vi "ActionController.vi"(0 "Error In":errorcluster, 5 "Water":dbl, 7 "Sound":dbl, 9 "on/off toggle":bool, 11 "direction toggle 2":bool) -> (4 "Error Out":errorcluster, 6 "감속":bool, 8 "LCD 변경":bool)   [LabVIEW 2019]
uses:
  LINE_2.vi
  LINE_1.vi
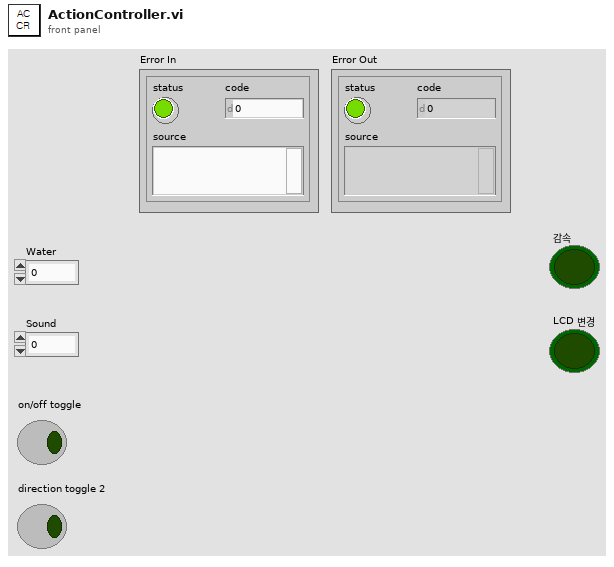
[diagram p1: front panel]
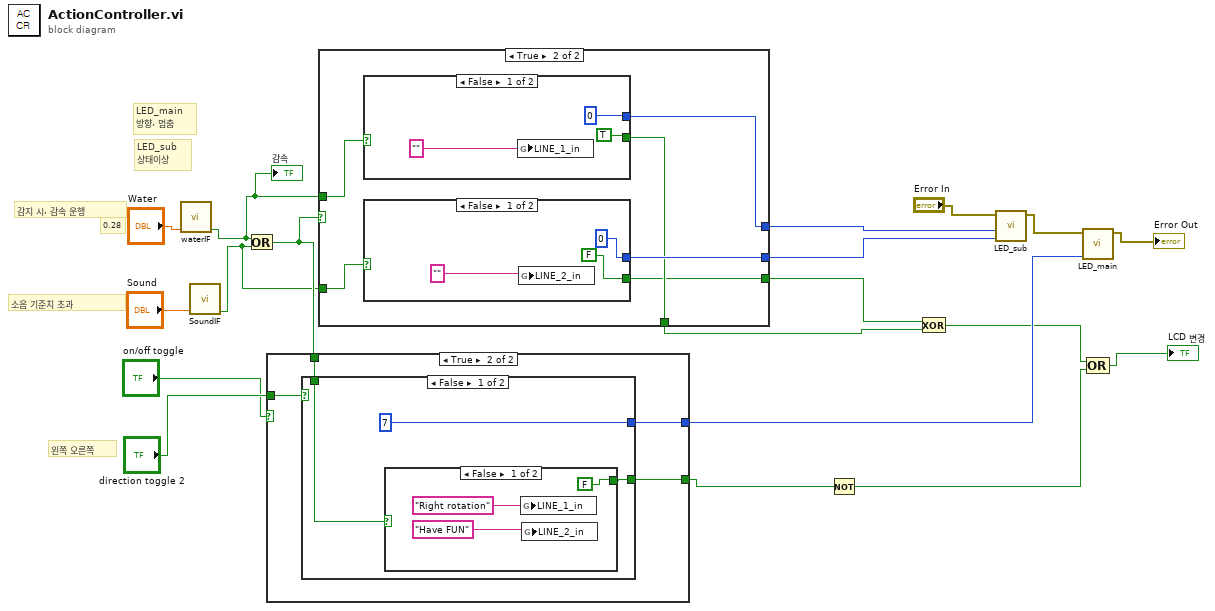
[diagram p0: block diagram]
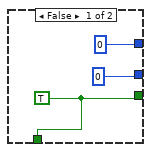
[diagram p2: hidden frame]
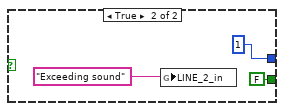
[diagram p3: hidden frame]
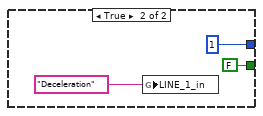
[diagram p4: hidden frame]
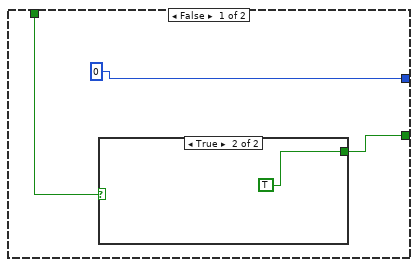
[diagram p5: hidden frame]
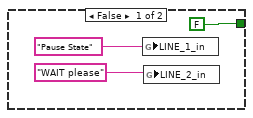
[diagram p6: hidden frame]
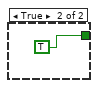
[diagram p7: hidden frame]
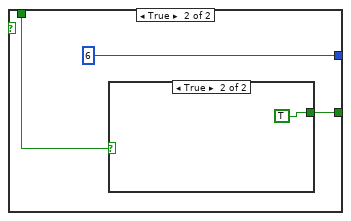
[diagram p8: hidden frame]
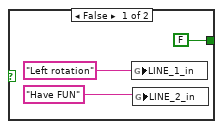
[diagram p9: hidden frame]
diagram:
  # "LED_sub\n상태이상"
  # "LED_main\n방향, 멈춤"
  # "왼쪽 오른쪽"
  # "소음 기준치 초과"
  # "감지 시, 감속 운행"
  # "0.28"
  n1 = call "waterIF.vi"("Numeric"="Water") -> ("Boolean"=w10:bool)  [unwired: 10 in]
  "감속" <- w10
  n2 = call "SoundIF.vi"("Numeric"="Sound") -> ("Boolean"=w13:bool)  [unwired: 10 in]
  n3 = Or(x=w10, y=w13) -> (x .or. y?=w14:bool)
  n4 = case shown="True" "on/off toggle" {
    tunnel: "direction toggle 2" -> [_ w30]
    tunnel: [0 w29] -> w15
    tunnel: w14 -> [w21 w28]
    tunnel: [w20 w27] -> w2
    frame False {
      n5 = case shown="True" w21 {
        tunnel: [FALSE TRUE] -> w20
        frame False {
          n6 = global write "LINE_1.vi" "LINE_1_in"("Pause State") -> ()
          n7 = global write "LINE_2.vi" "LINE_2_in"("WAIT please") -> ()
        }
        frame True {
        }
      }
    }
    frame True {
      n8 = case shown="False" w30 {
        tunnel: [7 6] -> w29
        tunnel: w28 -> [w32 w39]
        tunnel: [w31 w38] -> w27
        frame False {
          n9 = case shown="False" w32 {
            tunnel: [FALSE TRUE] -> w31
            frame False {
              n10 = global write "LINE_1.vi" "LINE_1_in"("Right rotation") -> ()
              n11 = global write "LINE_2.vi" "LINE_2_in"("Have FUN") -> ()
            }
            frame True {
            }
          }
        }
        frame True {
          n12 = case shown="True" w39 {
            tunnel: [FALSE TRUE] -> w38
            frame False {
              n13 = global write "LINE_1.vi" "LINE_1_in"("Left rotation") -> ()
              n14 = global write "LINE_2.vi" "LINE_2_in"("Have FUN") -> ()
            }
            frame True {
            }
          }
        }
      }
    }
  }
  n15 = case shown="True" w14 {
    tunnel: [0 w51] -> w12
    tunnel: w10 -> [_ w53]
    tunnel: w13 -> [_ w52]
    tunnel: [0 w50] -> w11
    tunnel: [w45 w49] -> w4
    tunnel: [w45 w48] -> w5
    frame False {
      w45 = TRUE
    }
    frame True {
      n16 = case shown="False" w53 {
        tunnel: [0 1] -> w51
        tunnel: [TRUE FALSE] -> w49
        frame False {
          n17 = global write "LINE_1.vi" "LINE_1_in"("") -> ()
        }
        frame True {
          n18 = global write "LINE_1.vi" "LINE_1_in"("Deceleration") -> ()
        }
      }
      n19 = case shown="False" w52 {
        tunnel: [0 1] -> w50
        tunnel: [FALSE FALSE] -> w48
        frame False {
          n20 = global write "LINE_2.vi" "LINE_2_in"("") -> ()
        }
        frame True {
          n21 = global write "LINE_2.vi" "LINE_2_in"("Exceeding sound") -> ()
        }
      }
    }
  }
  n22 = Not(x=w2) -> (.not. x?=w1:bool)
  n23 = Exclusive Or(1:w4, 2:w5) -> (0:w3:bool)
  n24 = call "LED_sub.vi"("sound"=w11, "water"=w12, "Error In"="Error In") -> ("Error Out"=w8:errorcluster)  [unwired: 8 in]
  n25 = call "LED_main.vi"("Numeric"=w15, "Error In"=w8) -> ("Error Out"=→"Error Out":errorcluster)  [unwired: 9 in]
  n26 = Compound Arithmetic op=OR(w3, w1) -> (→"LCD 변경":bool)
